vi "Get ECU Frame Indices.vi"(8 "error in":errorcluster, 10 "Frames":T1[](array[typedef]), 11 "XNET Frames":refnum<k21>[](array[refnum])) -> (0 "error out":errorcluster, 3 "Frame Indices":u32[](array[numeric]))   [LabVIEW 2020, in "Communication Bus Template System Explorer.lvlib" / "Implementation.lvlib"]
uses:
  Implementation.lvlib
  <resource>/objmgr/xnet.rc
  Types/Signal.ctl
  Types/Frame.ctl
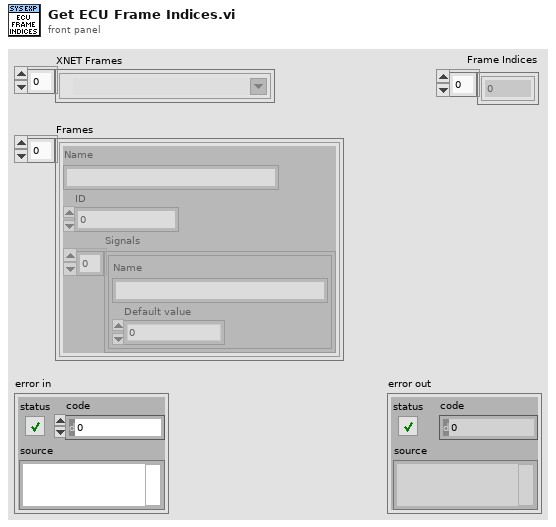
[diagram p1: front panel]
types:
  T1 = typedef "Communication Bus Template System Explorer.lvlib/Implementation.lvlib/Frame.ctl" = cluster{"Name":string, "ID":u32, "Signals":cluster{"Name":T2, "Default value":dbl}[]}
  T2 = typedef "Communication Bus Template System Explorer.lvlib/Implementation.lvlib/Signal.ctl" = string
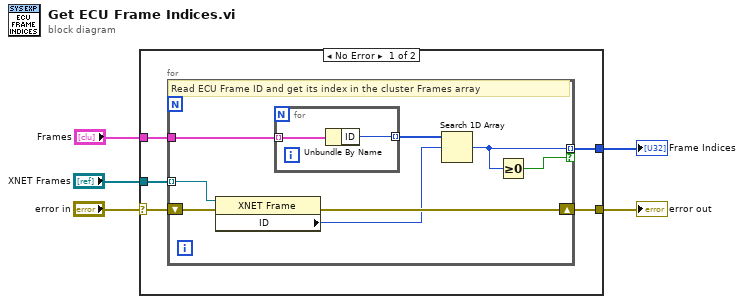
[diagram p0: block diagram]
diagram:
  n1 = case shown="No Error" "error in" {
    selector: "error in" -> [w8 w21]
    tunnel: "XNET Frames" -> [w10 _]
    tunnel: [w9 w21] -> w4
    tunnel: "Frames" -> [w7 _]
    tunnel: [w6 _] -> w1
    frame No Error {
      n2 = for {
        tunnel: w10 -> [w18] mode=indexing
        shift-right: [w16] -> w9
        shift-left: w8 -> [w17]
        tunnel: w7 -> [w13]
        tunnel: [w15] -> w6 mode=indexing if=w14
        # "Read ECU Frame ID and get its index in the cluster Frames array"
        n3 = property class="XNET Frame"(reference=w18, error in=w17) -> (error out=w16:errorcluster, "ID"=w11:u32)  [unwired: 1 out]
        n4 = for {
          tunnel: w13 -> [w20] mode=indexing
          tunnel: [w19] -> w12 mode=indexing
          n5 = Unbundle By Name(w20) -> ("ID"=w19:u32)
        }
        n6 = Search 1D Array(1D array=w12, element=w11) -> (index of element=w15:i32)  [unwired: 1 in]
        n7 = Greater Or Equal To 0?(x=w15) -> (x >= 0?=w14:bool)
      }
    }
    frame Error {
    }
  }
  "error out" <- w4
  "Frame Indices" <- w1
